vi "grayScale.vi"() -> ()   [LabVIEW 2023]
uses:
  <vilib>/vision/NI_Vision_Development_Module.lvlib
panel:
  out "Image Out 5":T1(plugin-control)
  out "Image Out 4":T1(plugin-control)
  in  "Range":cluster{"Lower value":sgl, "Upper value":sgl}={"Lower value"=128.0, "Upper value"=255.0} {"Upper value" format="%.2f"; "Lower value" format="%.2f"}
  out "Image Out 3":T1(plugin-control)
  out "Image Out 2":T1(plugin-control)
  in  "stop":bool
  out "Image Out":T1(plugin-control)
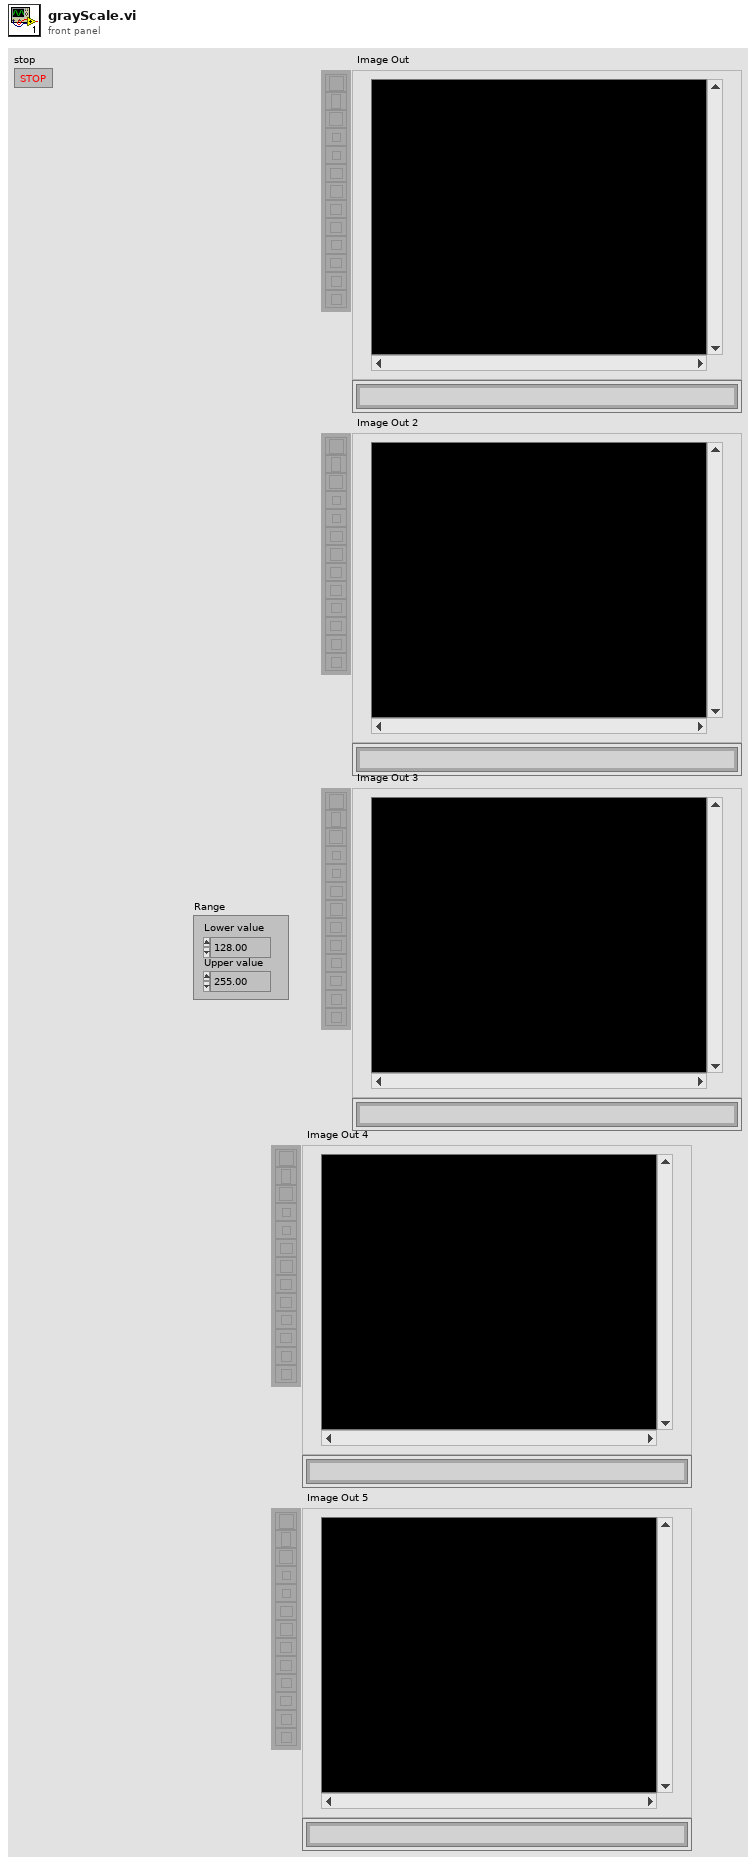
[diagram p1: front panel]
types:
  T1 = typedef "IMAQ Image.ctl" = refnum<image>
  T2 = typedef "Image Type" = u32
  T3 = typedef "Particle Parameters" = i32
  T4 = cluster{"Measurement Parameter":T3, "Range Lower Value":dbl, "Range Upper Value":dbl, "Range":bool, "Measurement Type":bool}[]
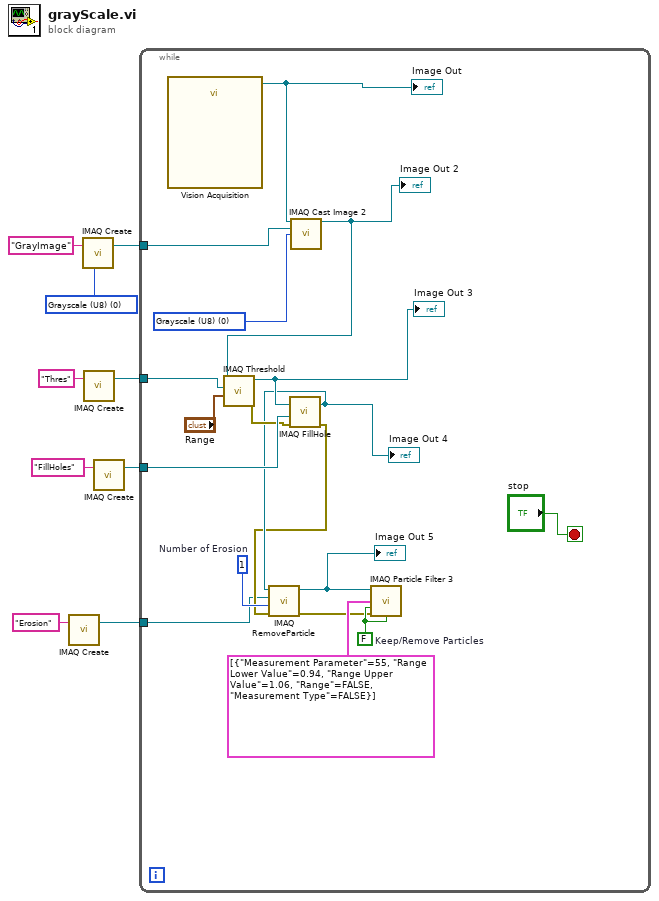
[diagram p0: block diagram]
diagram:
  w9 = T2 0 items=["Grayscale (U8)", "Grayscale (I16)", "Grayscale (SGL)", "Complex (CSG)", "RGB (U32)", "HSL (U32)", "RGB (U64)", "Grayscale (U16)"] ("Image Type")
  n1 = call "IMAQ Create"("Image Name"="Erosion") -> ("New Image"=w1:T1)  [unwired: 4 in, 1 out]
  n2 = call "IMAQ Create"("Image Name"="GrayImage", "Image Type"=w9) -> ("New Image"=w7:T1)  [unwired: 3 in, 1 out]
  n3 = call "IMAQ Create"("Image Name"="Thres") -> ("New Image"=w5:T1)  [unwired: 4 in, 1 out]
  n4 = call "IMAQ Create"("Image Name"="FillHoles") -> ("New Image"=w3:T1)  [unwired: 4 in, 1 out]
  n5 = while {
    tunnel: w7 -> [w25]
    tunnel: w5 -> [w23]
    tunnel: w3 -> [w19]
    tunnel: w1 -> [w10]
    stop <- "stop" stop-if-true
    w15 = 1  # Number of Erosion
    w17 = FALSE  # Keep/Remove Particles
    w26 = T2 0 items=["Grayscale (U8)", "Grayscale (I16)", "Grayscale (SGL)", "Complex (CSG)", "RGB (U32)", "HSL (U32)", "RGB (U64)", "Grayscale (U16)"] ("Image Type")
    n6 = call "Vision Acquisition"() -> ("Image Out"=w24:T1)  [unwired: 25 in, 2 out]
    "Image Out" <- w24
    n7 = call "IMAQ Cast Image 2"("Image Src"=w24, "Image Dst"=w25, "Image Type"=w26) -> ("Image Dst Out"=w22:T1)  [unwired: 11 in, 1 out]
    "Image Out 2" <- w22
    n8 = call "IMAQ Threshold"("Range"="Range", "Image Dst"=w23, "Image Src"=w22) -> ("error out"=w18:errorcluster, "Image Dst Out"=w20:T1)  [unwired: 7 in]
    "Image Out 3" <- w20
    n9 = call "IMAQ FillHole"("error in (no error)"=w18, "Image Dst"=w19, "Image Src"=w20) -> ("error out"=w12:errorcluster, "Image Dst Out"=w13:T1)  [unwired: 3 in]
    "Image Out 4" <- w13
    n10 = call "IMAQ RemoveParticle"("error in (no error)"=w12, "Number of Erosion"=w15, "Image Dst"=w10, "Image Src"=w13) -> ("error out"=w14:errorcluster, "Image Dst Out"=w11:T1)  [unwired: 6 in]
    "Image Out 5" <- w11
    n11 = call "IMAQ Particle Filter 3"("Image Src"=w11, "Selection Values"=T4 [{"Measurement Parameter"=55, "Range Lower Value"=0.94, "Range Upper Value"=1.06, "Range"=FALSE, "Measurement Type"=FALSE}], "Keep/Remove Particles (F)"=w17, "error in (no error)"=w14, "Fill Holes? (F)"=w17) -> ()  [unwired: 8 in, 3 out]
  }
